vi "超标留样留样命令.vi"(8 "error in (no error)":errorcluster) -> (0 "error out":errorcluster)   [LabVIEW 2016, in "科盛超标留样.lvlib"]
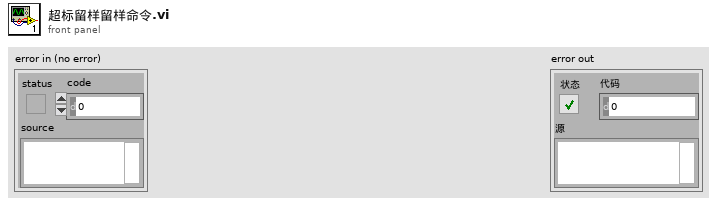
[diagram p1: front panel]
types:
  T1 = cluster{"STEP":enum16{"open", "read", "write", "close"}, "写入缓冲区":string}
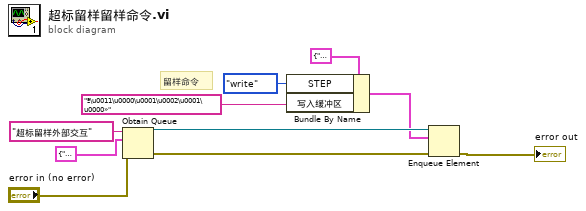
[diagram p0: block diagram]
diagram:
  # "留样命令"
  n1 = Obtain Queue(name (unnamed)="超标留样外部交互" ("名称（未命名）"), element data type=T1 {"STEP"=enum."write", "写入缓冲区"="ª\u0006\u0000\u0000P`\u00000»"}, error in (no error)="error in (no error)") -> (queue out=w8:refnum<queue>, error out=w7:errorcluster)  [unwired: 2 in, 1 out]
  n2 = Bundle By Name(cluster=T1 {"STEP"=enum."open", "写入缓冲区"=""} ("元素"), "STEP"=enum16{"open", "read", "write", "close"}."write", "写入缓冲区"="ª\u0011\u0000\u0001\u0002\u0001\u0000»") -> (w4:T1)
  n3 = Enqueue Element(queue=w8, element=w4, error in (no error)=w7) -> (error out=→"error out":errorcluster)  [unwired: 1 in, 2 out]
